vi "niLvFpga_ConfigureFifo_cRIO-9046.vi"(0 "session in":u32, 5 "channel":u32=1, 7 "Fifo Depth":u32, 11 "error in (no error)":errorcluster) -> (4 "session out":u32, 8 "actualDepth":u32, 15 "error out":errorcluster)   [LabVIEW 2020]
uses:
  NiFpgaLv.dll
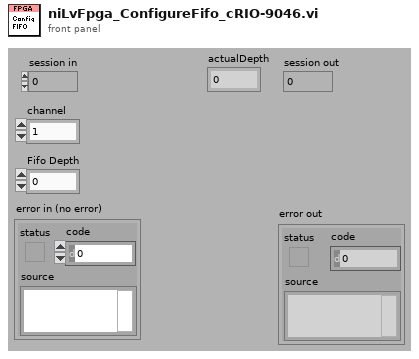
[diagram p1: front panel]
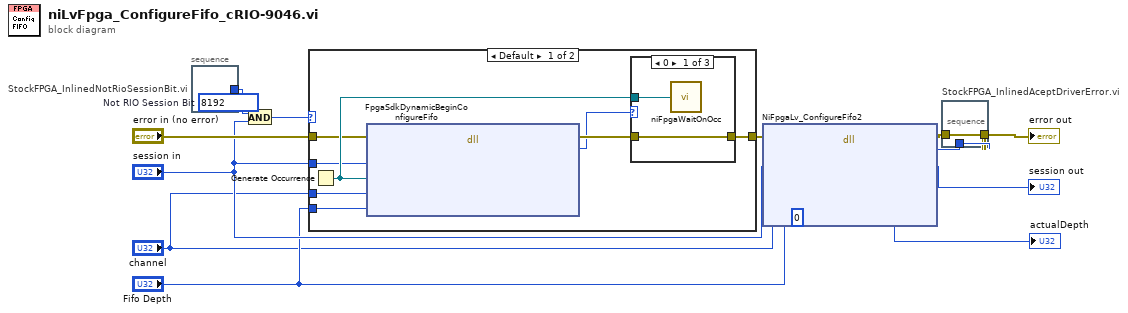
[diagram p0: block diagram]
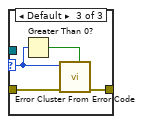
[diagram p4: hidden frame]
diagram:
  n1 = stacked-sequence "StockFPGA_InlinedNotRioSessionBit.vi" {
    tunnel: [w14] -> w9
    frame #0 {
      w14 = u32 8192  # Not RIO Session Bit
    }
  }
  n2 = And(x=w9, y="session in") -> (x .and. y?=w8:u32)
  n3 = case shown="Default" w8 {
    tunnel: "error in (no error)" -> [w19 w30]
    tunnel: [w18 w30] -> w6
    tunnel: "session in" -> [w17 _]
    tunnel: "channel" -> [w16 _]
    tunnel: "Fifo Depth" -> [w15 _]
    frame Default {
      n4 = Generate Occurrence() -> (w22:refnum<k4>)
      n5 = dll-call lib="LabVIEW" fn="FpgaSdkDynamicBeginConfigureFifo"(error in=w19, "session"=w17, "occurrence"=w22, "channel"=w16, "fifoDepth"=w15) -> (error out=w21:errorcluster, "status"=w20:i32)  [unwired: 6 in, 1 out]
      n6 = case shown="0" w20 {
        selector: w20 -> [_ _ w26]
        tunnel: [w24 w25 w28] -> w18
        tunnel: w21 -> [w24 w25 w29]
        tunnel: w22 -> [w23 _ _]
        frame 0 {
          n7 = call <vilib>:"niFpgaWaitOnOcc.vi"("occurrence"=w23) -> ()  [unwired: 14 in, 1 out]
        }
        frame -61167 {
          # "emulation case intentionally ignoring error"
        }
        frame Default {
          n8 = Greater Than 0?(x=w26) -> (x > 0?=w27:bool)
          n9 = call <vilib>:"Error Cluster From Error Code.vi"("is warning? (False)"=w27, "error in (no error)"=w29, "error code (0)"=w26) -> ("error out"=w28:errorcluster)  [unwired: 6 in]
        }
      }
    }
    frame 0 {
    }
  }
  n10 = dll-call lib="NiFpgaLv.*" fn="NiFpgaLv_ConfigureFifo2" label="niLvFpgaConfigureFifo"(error in=w6, "sessionID"="session in", "channel"="channel", "fifoDepth"="Fifo Depth", "actualDepth"=u32 0) -> (error out=w12:errorcluster, "status"=w10:i32, "sessionID"=→"session out":u32, "actualDepth"=→"actualDepth":u32)  [unwired: 4 in, 1 out]
  n11 = stacked-sequence "StockFPGA_InlinedAceptDriverError.vi" {
    tunnel: w12 -> [w31]
    tunnel: w10 -> [w33]
    tunnel: [w32] -> w11
    frame #0 {
      n12 = case shown="Default" w33 {
        selector: w33 -> [_ w35]
        tunnel: [w34 w37] -> w32
        tunnel: w31 -> [w34 w38]
        frame 0 {
        }
        frame Default {
          n13 = Greater Than 0?(x=w35) -> (x > 0?=w36:bool)
          n14 = call <vilib>:"Error Cluster From Error Code.vi"("is warning? (False)"=w36, "error in (no error)"=w38, "error code (0)"=w35) -> ("error out"=w37:errorcluster)  [unwired: 6 in]
        }
      }
    }
  }
  "error out" <- w11
